vi "read data from lard.vi"() -> (0 "pos x":i16, 3 "distance":fxp<+/-,32,16>[](array[numeric]), 4 "pos y":i16, 6 "heading":i16)   [LabVIEW 2014]
uses:
  Robot Global Data.vi
panel:
  out "pos x 2":i16
  out "pos y 2":i16
  out "heading 2":sgl
  out "distance 2":fxp<+/-,32,16>[](array[numeric])
  in  "Boolean 2":bool
  in  "Boolean":bool
  out "Received Data":u8[](array[numeric])
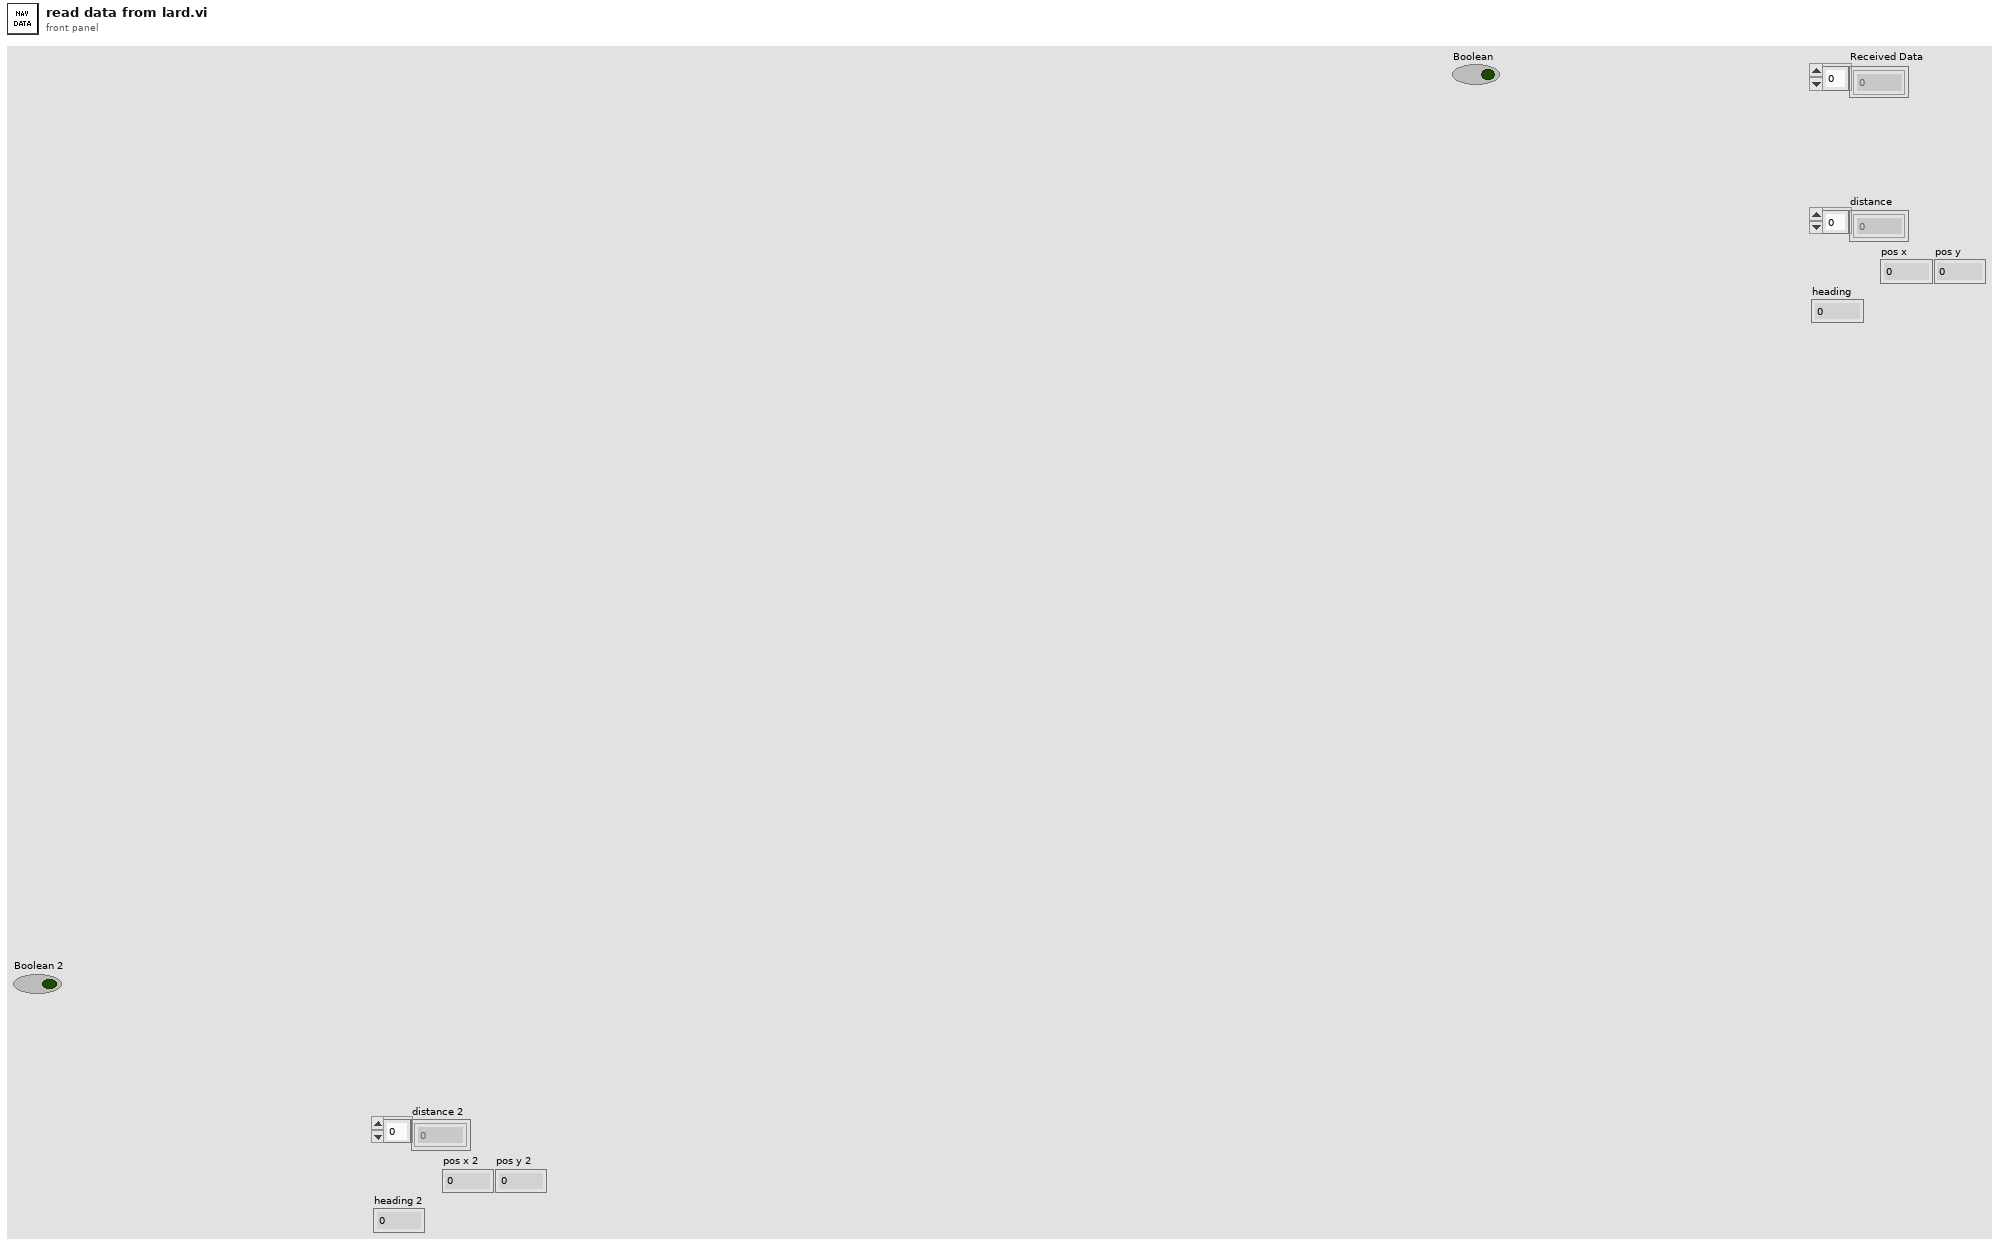
[diagram p1: front panel]
types:
  T1 = typedef "WPI_SerialPortRef.ctl" = cluster{"DevStatus":errorcluster, "Serial Port Name":refnum<visa-resource-name>}
  T2 = typedef "WPI_SPIDevRef.ctl" = cluster{"DevStatus":errorcluster, "Handle":i32, "Controller":T3, "SPI Bus":T4}
  T3 = typedef "FPGA_TypedefDigitalModule.ctl" = enum16{"Controller 1"}
  T4 = typedef "spi_bus.ctl" = enum16{"SPI On-Board, CS0", "SPI On-Board, CS1", "SPI On-Board, CS2", "SPI On-Board, CS3", "SPI MXP", "Invalid"}
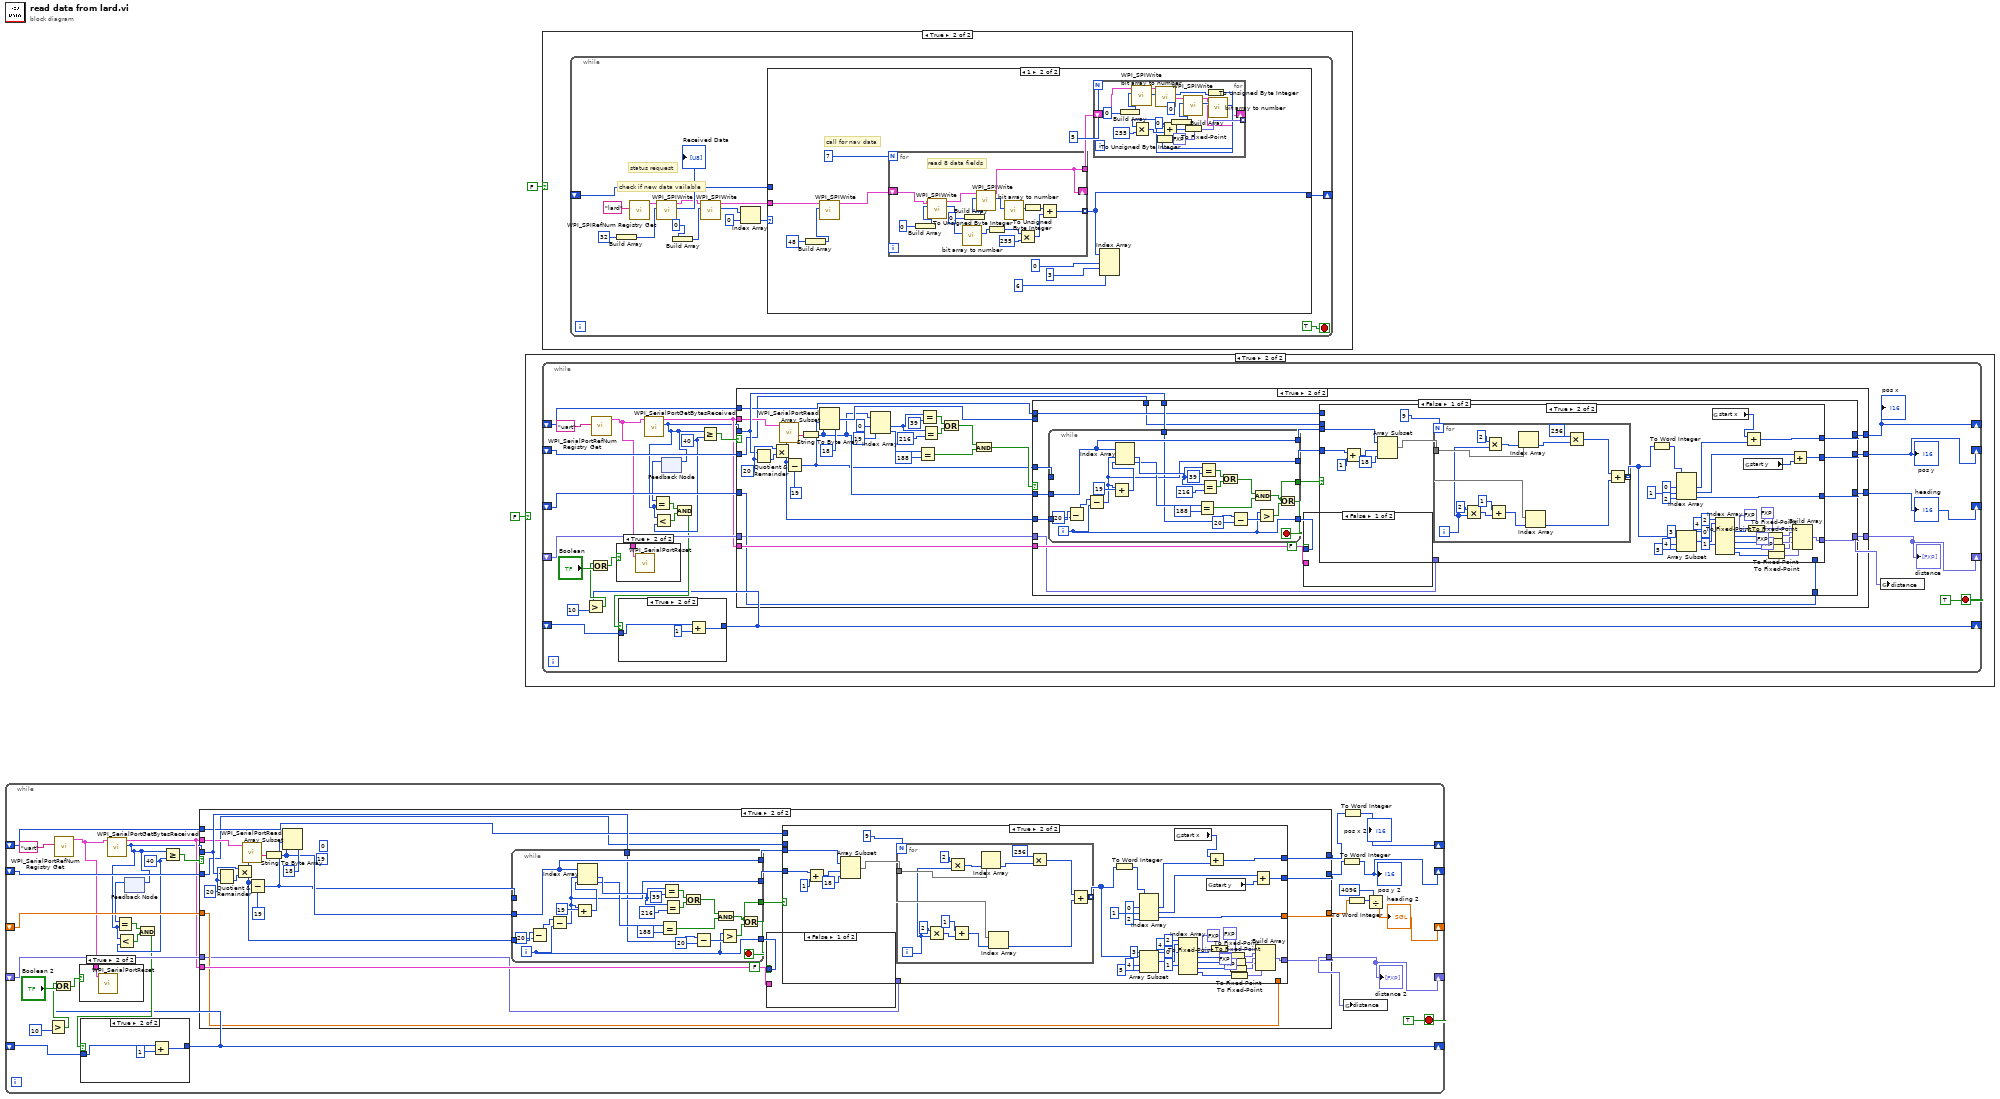
[diagram p0: block diagram]
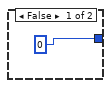
[diagram p2: hidden frame]
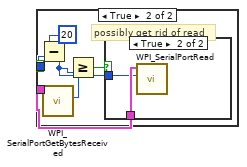
[diagram p6: hidden frame]
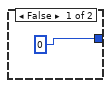
[diagram p9: hidden frame]
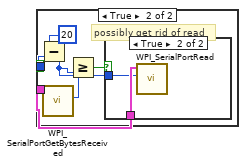
[diagram p13: hidden frame]
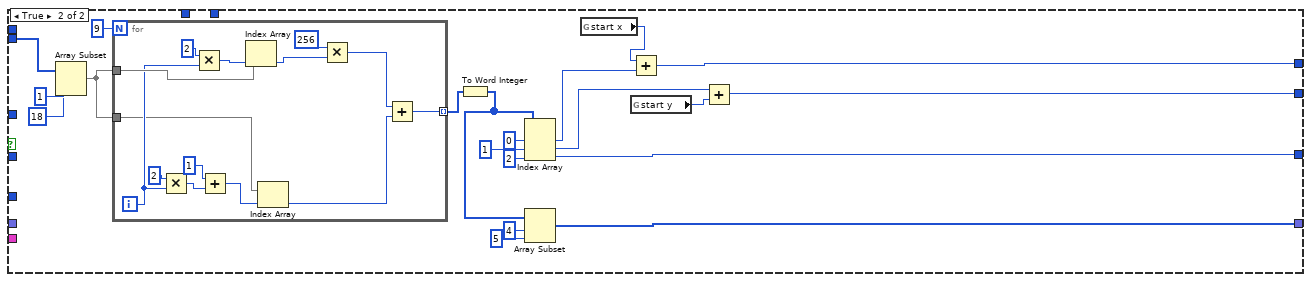
[diagram p15: hidden frame]
diagram:
  n1 = while {
    shift-right: [w9] -> _
    shift-left: _ -> [w29]
    shift-right: [w7] -> _
    shift-left: _ -> [w28]
    shift-right: [w3] -> _
    shift-left: _ -> [w27]
    shift-right: [w25] -> _
    shift-left: _ -> [w26]
    shift-right: [w11] -> _
    shift-left: _ -> [w14]
    stop <- TRUE stop-if-true
    w18 = u32 40 ("y")
    n2 = call <vilib>:"WPI_SerialPortRefNum Registry Get.vi"("refnum name"="uart") -> ("SerialPortRef"=w23:T1)  [unwired: 9 in, 1 out]
    n3 = call <vilib>:"WPI_SerialPortGetBytesReceived.vi"("SerialPortRef"=w23) -> ("Bytes at Port"=w19:u32, "SerialPortRef"=w24:T1)  [unwired: 8 in, 1 out]
    n4 = Less?(x=w19, y=w18) -> (x < y?=w16:bool)
    n5 = feedback-in #1(w19) -> ()
    n6 = feedback #1() -> (w20:u32)  [unwired: 1 in]
    n7 = Equal?(x=w20, y=w19) -> (x = y?=w17:bool)
    n8 = And(x=w17, y=w16) -> (x .and. y?=w15:bool)
    n9 = case shown="True" w15 {
      tunnel: [0 w34] -> w11
      tunnel: w14 -> [_ w36]
      frame False {
      }
      frame True {
        n10 = Add(x=w36, y=1) -> (x+y=w34:i32)
      }
    }
    n11 = Greater?(x=w11, y=10) -> (0:w12:bool)
    n12 = Or(x=w12, y="Boolean 2") -> (x .or. y?=w22:bool)
    n13 = case shown="True" w22 {
      tunnel: w23 -> [_ w37]
      frame False {
      }
      frame True {
        n14 = call <vilib>:"WPI_SerialPortReset.vi"("SerialPortRef"=w37) -> ()  [unwired: 9 in, 2 out]
      }
    }
    n15 = Greater Or Equal?(x=w19, y=w18) -> (x >= y?=w31:bool)
    n16 = case shown="True" w31 {
      tunnel: w24 -> [_ w51]
      tunnel: w19 -> [_ w52]
      tunnel: [w41 w62] -> w10
      tunnel: [w40 w61] -> w8
      tunnel: [w39 w60] -> w6
      tunnel: [w38 w59] -> w25
      tunnel: w29 -> [w41 w50]
      tunnel: w28 -> [w40 w49]
      tunnel: w27 -> [w39 w48]
      tunnel: w26 -> [w38 w47]
      tunnel: w24 -> [_ w55]
      frame False {
      }
      frame True {
        (unwired) 19 ("index")
        (unwired) 0 ("index")
        w58 = u32 20 ("y")
        n17 = Quotient & Remainder(x=w52, y=w58) -> (floor(x/y)=w57:u32)  [unwired: 1 out]
        n18 = Multiply(x=w58, y=w57) -> (x*y=w56:u32)
        n19 = call <vilib>:"WPI_SerialPortRead.vi"("Num Bytes to Read"=w56, "SerialPortRef"=w51) -> ("Buffer"=w65:string)  [unwired: 7 in, 2 out]
        n20 = Subtract(x=w56, y=u32 19) -> (x-y=w53:u32)
        n21 = String To Byte Array(string=w65) -> (unsigned byte array=w54:u8[])
        n22 = Array Subset(array=w54, index=w53, length=18) -> ()  [unwired: 1 out]
        n23 = while {
          tunnel: w54 -> [w146]
          tunnel: w56 -> [w138]
          tunnel: [w146] -> w46
          tunnel: [w139] -> w45
          tunnel: w53 -> [_]
          tunnel: [w143] -> w44
          tunnel: w52 -> [w142]
          tunnel: [w134] -> w42
          i -> [w139]
          stop <- w147 stop-if-true
          n24 = Subtract(x=w138, y=u32 20) -> (x-y=w136:u32)
          n25 = Subtract(x=w136, y=w139) -> (x-y=w143:u32)
          n26 = Add(x=w143, y=u32 19) -> (x+y=w144:u32)
          n27 = Index Array(array=w146, index #1=w143, index #2=w144) -> (element #1=w149:u8, element #2=w148:u8)
          n28 = Equal?(x=w148, y=u8 188) -> (x = y?=w150:bool)
          n29 = Equal?(x=w149, y=u8 39) -> (x = y?=w153:bool)
          n30 = Equal?(x=w149, y=u8 216) -> (x = y?=w152:bool)
          n31 = Or(x=w153, y=w152) -> (x .or. y?=w151:bool)
          n32 = Subtract(x=w142, y=u32 20) -> (x-y=w140:u32)
          n33 = And(x=w151, y=w150) -> (x .and. y?=w134:bool)
          n34 = Greater?(x=w139, y=w140) -> (0:w135:bool)
          n35 = Or(x=w134, y=w135) -> (x .or. y?=w147:bool)
        }
        n36 = case shown="False" FALSE {
          tunnel: w45 -> [_ w128]
          tunnel: w55 -> [_ w127]
          frame False {
          }
          frame True {
            # "possibly get rid of read"
            n37 = Subtract(x=20, y=w128) -> (x-y=w126:i32)
            n38 = call <vilib>:"WPI_SerialPortGetBytesReceived.vi"("SerialPortRef"=w127) -> ("Bytes at Port"=w130:u32)  [unwired: 8 in, 2 out]
            n39 = Greater Or Equal?(x=w130, y=w126) -> (x >= y?=w131:bool)
            n40 = case shown="True" w131 {
              tunnel: w127 -> [_ w133]
              tunnel: w126 -> [_ w132]
              frame False {
              }
              frame True {
                n41 = call <vilib>:"WPI_SerialPortRead.vi"("Num Bytes to Read"=w132, "SerialPortRef"=w133) -> ()  [unwired: 7 in, 3 out]
              }
            }
          }
        }
        n42 = case shown="True" w42 {
          tunnel: w46 -> [_ w103]
          tunnel: [w69 w98] -> w62
          tunnel: [w68 w97] -> w61
          tunnel: [w67 w96] -> w60
          tunnel: [w66 w70] -> w59
          tunnel: w44 -> [_ w93]
          tunnel: w50 -> [w69 _]
          tunnel: w49 -> [w68 _]
          tunnel: w48 -> [w67 _]
          tunnel: w47 -> [w66 _]
          frame False {
          }
          frame True {
            n43 = Add(x=w93, y=u32 1) -> (x+y=w102:u32)
            n44 = Array Subset(array=w103, index=w102, length=18) -> (w100:u8[])
            n45 = for {
              N: 9 -> [_]
              tunnel: w100 -> [w115]
              tunnel: [w113] -> w95 mode=indexing
              i -> [w114]
              n46 = Multiply(x=2, y=w114) -> (x*y=w122:i32)
              n47 = Multiply(x=2, y=w114) -> (x*y=w125:i32)
              n48 = Add(x=1, y=w122) -> (x+y=w120:i32)
              n49 = Index Array(array=w115, index=w125) -> (element=w118:u8)
              n50 = Index Array(array=w115, index=w120) -> (element=w116:u8)
              n51 = Multiply(x=i16 256, y=w118) -> (x*y=w117:i16)
              n52 = Add(x=w117, y=w116) -> (x+y=w113:i16)
            }
            n53 = To Word Integer(number=w95) -> (16bit integer=w94:i16[])
            n54 = Index Array(array=w94, index #1=0 ("index"), index #2=1 ("index"), index #3=2 ("index")) -> (element #1=w107:i16, element #2=w106:i16, element #3=w96:i16)
            n55 = Array Subset(array=w95, index=4, length=5) -> (w90:i16[])
            n56 = global read "Robot Global Data.vi" "start x"() -> (w109:u16)
            n57 = Index Array(array=w90, index #1=0 ("index"), index #2=1 ("index"), index #3=2 ("index"), index #4=3 ("index"), index #5=4 ("index")) -> (element #1=w88:i16, element #2=w85:i16, element #3=w84:i16, element #4=w81:i16, element #5=w80:i16)
            n58 = Add(x=w109, y=w107) -> (x+y=w98:u16)
            n59 = global read "Robot Global Data.vi" "start y"() -> (w108:u16)
            n60 = To Fixed-Point(fixed-point type=fxp<+/-,32,16> 8.0, number=w88) -> (fixed-point=w75:fxp<+/-,32,16>)
            n61 = To Fixed-Point(fixed-point type=fxp<+/-,32,16> 8.0, number=w85) -> (fixed-point=w74:fxp<+/-,32,16>)
            n62 = To Fixed-Point(fixed-point type=fxp<+/-,32,16> 8.0, number=w84) -> (fixed-point=w73:fxp<+/-,32,16>)
            n63 = To Fixed-Point(fixed-point type=fxp<+/-,32,16> 8.0, number=w81) -> (fixed-point=w72:fxp<+/-,32,16>)
            n64 = To Fixed-Point(fixed-point type=fxp<+/-,32,16> 8.0, number=w80) -> (fixed-point=w71:fxp<+/-,32,16>)
            n65 = Add(x=w106, y=w108) -> (x+y=w97:u16)
            n66 = Build Array(w75, w74, w73, w72, w71) -> (w70:fxp<+/-,32,16>[])
          }
        }
      }
    }
    "distance 2" <- w25
    n67 = To Word Integer(number=w8) -> (16bit integer=w7:i16)
    "pos y 2" <- w7
    n68 = To Word Integer(number=w10) -> (16bit integer=w9:i16)
    "pos x 2" <- w9
    n69 = global write "Robot Global Data.vi" "distance"(w25) -> ()
    n70 = To Word Integer(number=w6) -> (16bit integer=w5:i16)
    n71 = Divide(x=w5, y=i16 4096) -> (x/y=w3:dbl)
    "heading 2" <- w3
  }
  n72 = case shown="True" FALSE {
    frame False {
    }
    frame True {
      n73 = while {
        shift-right: [w178] -> _
        shift-left: _ -> [w175]
        shift-right: [w177] -> _
        shift-left: _ -> [w174]
        shift-right: [w176] -> _
        shift-left: _ -> [w173]
        shift-right: [w171] -> _
        shift-left: _ -> [w172]
        shift-right: [w157] -> _
        shift-left: _ -> [w160]
        stop <- TRUE stop-if-true
        w164 = u32 40 ("y")
        n74 = call <vilib>:"WPI_SerialPortRefNum Registry Get.vi"("refnum name"="uart") -> ("SerialPortRef"=w169:T1)  [unwired: 9 in, 1 out]
        n75 = call <vilib>:"WPI_SerialPortGetBytesReceived.vi"("SerialPortRef"=w169) -> ("Bytes at Port"=w165:u32, "SerialPortRef"=w170:T1)  [unwired: 8 in, 1 out]
        n76 = Less?(x=w165, y=w164) -> (x < y?=w162:bool)
        n77 = feedback-in #2(w165) -> ()
        n78 = feedback #2() -> (w166:u32)  [unwired: 1 in]
        n79 = Equal?(x=w166, y=w165) -> (x = y?=w163:bool)
        n80 = And(x=w163, y=w162) -> (x .and. y?=w161:bool)
        n81 = case shown="True" w161 {
          tunnel: [0 w183] -> w157
          tunnel: w160 -> [_ w185]
          frame False {
          }
          frame True {
            n82 = Add(x=w185, y=1) -> (x+y=w183:i32)
          }
        }
        n83 = Greater?(x=w157, y=10) -> (0:w158:bool)
        n84 = Or(x=w158, y="Boolean") -> (x .or. y?=w168:bool)
        n85 = case shown="True" w168 {
          tunnel: w169 -> [_ w186]
          frame False {
          }
          frame True {
            n86 = call <vilib>:"WPI_SerialPortReset.vi"("SerialPortRef"=w186) -> ()  [unwired: 9 in, 2 out]
          }
        }
        n87 = Greater Or Equal?(x=w165, y=w164) -> (x >= y?=w180:bool)
        n88 = case shown="True" w180 {
          tunnel: w170 -> [_ w195]
          tunnel: w165 -> [_ w196]
          tunnel: [w190 w219] -> w178
          tunnel: [w189 w218] -> w177
          tunnel: [w188 w217] -> w176
          tunnel: [w187 w216] -> w171
          tunnel: w175 -> [w190 w194]
          tunnel: w174 -> [w189 w193]
          tunnel: w173 -> [w188 w192]
          tunnel: w172 -> [w187 w191]
          tunnel: w170 -> [_ w199]
          frame False {
          }
          frame True {
            w215 = u32 20 ("y")
            n89 = Quotient & Remainder(x=w196, y=w215) -> (floor(x/y)=w214:u32)  [unwired: 1 out]
            n90 = Multiply(x=w215, y=w214) -> (x*y=w200:u32)
            n91 = call <vilib>:"WPI_SerialPortRead.vi"("Num Bytes to Read"=w200, "SerialPortRef"=w195) -> ("Buffer"=w222:string)  [unwired: 7 in, 2 out]
            n92 = Subtract(x=w200, y=u32 19) -> (x-y=w197:u32)
            n93 = String To Byte Array(string=w222) -> (unsigned byte array=w198:u8[])
            n94 = Array Subset(array=w198, index=w197, length=18) -> (w201:u8[])
            n95 = Index Array(array=w198, index #1=0 ("index"), index #2=19 ("index")) -> (element #1=w210:u8, element #2=w208:u8)
            n96 = Equal?(x=w208, y=u8 188) -> (x = y?=w203:bool)
            n97 = Equal?(x=w210, y=u8 39) -> (x = y?=w206:bool)
            n98 = Equal?(x=w210, y=u8 216) -> (x = y?=w205:bool)
            n99 = Or(x=w206, y=w205) -> (x .or. y?=w204:bool)
            n100 = And(x=w204, y=w203) -> (x .and. y?=w202:bool)
            n101 = case shown="False" w202 {
              tunnel: [w237 w341] -> w219
              tunnel: [w236 w340] -> w218
              tunnel: [w235 w339] -> w217
              tunnel: [w234 w338] -> w216
              tunnel: w201 -> [_ w337]
              tunnel: w198 -> [w240 _]
              tunnel: w200 -> [w239 _]
              tunnel: w199 -> [w232 _]
              tunnel: w197 -> [w231 _]
              tunnel: w196 -> [w229 _]
              tunnel: w194 -> [w227 _]
              tunnel: w193 -> [w226 _]
              tunnel: w192 -> [w225 _]
              tunnel: w191 -> [w224 _]
              frame False {
                n102 = while {
                  tunnel: w240 -> [w321]
                  tunnel: w239 -> [w313]
                  tunnel: [w321] -> w238
                  tunnel: [w314] -> w233
                  tunnel: w231 -> [_]
                  tunnel: [w318] -> w230
                  tunnel: w229 -> [w317]
                  tunnel: [w309] -> w223
                  i -> [w314]
                  stop <- w322 stop-if-true
                  n103 = Subtract(x=w313, y=u32 20) -> (x-y=w311:u32)
                  n104 = Subtract(x=w311, y=w314) -> (x-y=w318:u32)
                  n105 = Add(x=w318, y=u32 19) -> (x+y=w319:u32)
                  n106 = Index Array(array=w321, index #1=w318, index #2=w319) -> (element #1=w324:u8, element #2=w323:u8)
                  n107 = Equal?(x=w323, y=u8 188) -> (x = y?=w325:bool)
                  n108 = Equal?(x=w324, y=u8 39) -> (x = y?=w328:bool)
                  n109 = Equal?(x=w324, y=u8 216) -> (x = y?=w327:bool)
                  n110 = Or(x=w328, y=w327) -> (x .or. y?=w326:bool)
                  n111 = Subtract(x=w317, y=u32 20) -> (x-y=w315:u32)
                  n112 = And(x=w326, y=w325) -> (x .and. y?=w309:bool)
                  n113 = Greater?(x=w314, y=w315) -> (0:w310:bool)
                  n114 = Or(x=w309, y=w310) -> (x .or. y?=w322:bool)
                }
                n115 = case shown="False" FALSE {
                  tunnel: w233 -> [_ w303]
                  tunnel: w232 -> [_ w302]
                  frame False {
                  }
                  frame True {
                    # "possibly get rid of read"
                    n116 = Subtract(x=20, y=w303) -> (x-y=w301:i32)
                    n117 = call <vilib>:"WPI_SerialPortGetBytesReceived.vi"("SerialPortRef"=w302) -> ("Bytes at Port"=w305:u32)  [unwired: 8 in, 2 out]
                    n118 = Greater Or Equal?(x=w305, y=w301) -> (x >= y?=w306:bool)
                    n119 = case shown="True" w306 {
                      tunnel: w302 -> [_ w308]
                      tunnel: w301 -> [_ w307]
                      frame False {
                      }
                      frame True {
                        n120 = call <vilib>:"WPI_SerialPortRead.vi"("Num Bytes to Read"=w307, "SerialPortRef"=w308) -> ()  [unwired: 7 in, 3 out]
                      }
                    }
                  }
                }
                n121 = case shown="True" w223 {
                  tunnel: w238 -> [_ w278]
                  tunnel: [w244 w273] -> w237
                  tunnel: [w243 w272] -> w236
                  tunnel: [w242 w271] -> w235
                  tunnel: [w241 w245] -> w234
                  tunnel: w230 -> [_ w268]
                  tunnel: w227 -> [w244 _]
                  tunnel: w226 -> [w243 _]
                  tunnel: w225 -> [w242 _]
                  tunnel: w224 -> [w241 _]
                  frame False {
                  }
                  frame True {
                    n122 = Add(x=w268, y=u32 1) -> (x+y=w277:u32)
                    n123 = Array Subset(array=w278, index=w277, length=18) -> (w275:u8[])
                    n124 = for {
                      N: 9 -> [_]
                      tunnel: w275 -> [w290]
                      tunnel: [w288] -> w270 mode=indexing
                      i -> [w289]
                      n125 = Multiply(x=2, y=w289) -> (x*y=w297:i32)
                      n126 = Multiply(x=2, y=w289) -> (x*y=w300:i32)
                      n127 = Add(x=1, y=w297) -> (x+y=w295:i32)
                      n128 = Index Array(array=w290, index=w300) -> (element=w293:u8)
                      n129 = Index Array(array=w290, index=w295) -> (element=w291:u8)
                      n130 = Multiply(x=i16 256, y=w293) -> (x*y=w292:i16)
                      n131 = Add(x=w292, y=w291) -> (x+y=w288:i16)
                    }
                    n132 = To Word Integer(number=w270) -> (16bit integer=w269:i16[])
                    n133 = Index Array(array=w269, index #1=0 ("index"), index #2=1 ("index"), index #3=2 ("index")) -> (element #1=w282:i16, element #2=w281:i16, element #3=w271:i16)
                    n134 = Array Subset(array=w270, index=4, length=5) -> (w265:i16[])
                    n135 = global read "Robot Global Data.vi" "start x"() -> (w284:u16)
                    n136 = Index Array(array=w265, index #1=0 ("index"), index #2=1 ("index"), index #3=2 ("index"), index #4=3 ("index"), index #5=4 ("index")) -> (element #1=w263:i16, element #2=w260:i16, element #3=w259:i16, element #4=w256:i16, element #5=w255:i16)
                    n137 = Add(x=w284, y=w282) -> (x+y=w273:u16)
                    n138 = global read "Robot Global Data.vi" "start y"() -> (w283:u16)
                    n139 = To Fixed-Point(fixed-point type=fxp<+/-,32,16> 8.0, number=w263) -> (fixed-point=w250:fxp<+/-,32,16>)
                    n140 = To Fixed-Point(fixed-point type=fxp<+/-,32,16> 8.0, number=w260) -> (fixed-point=w249:fxp<+/-,32,16>)
                    n141 = To Fixed-Point(fixed-point type=fxp<+/-,32,16> 8.0, number=w259) -> (fixed-point=w248:fxp<+/-,32,16>)
                    n142 = To Fixed-Point(fixed-point type=fxp<+/-,32,16> 8.0, number=w256) -> (fixed-point=w247:fxp<+/-,32,16>)
                    n143 = To Fixed-Point(fixed-point type=fxp<+/-,32,16> 8.0, number=w255) -> (fixed-point=w246:fxp<+/-,32,16>)
                    n144 = Add(x=w281, y=w283) -> (x+y=w272:u16)
                    n145 = Build Array(w250, w249, w248, w247, w246) -> (w245:fxp<+/-,32,16>[])
                  }
                }
              }
              frame True {
                n146 = Array Subset(array=w337, index=1, length=18) -> (w334:u8[])
                n147 = for {
                  N: 9 -> [_]
                  tunnel: w334 -> [w363]
                  tunnel: w334 -> [w357]
                  tunnel: [w352] -> w333 mode=indexing
                  i -> [w362]
                  n148 = Multiply(x=2, y=w362) -> (x*y=w360:i32)
                  n149 = Multiply(x=2, y=w362) -> (x*y=w365:i32)
                  n150 = Add(x=1, y=w360) -> (x+y=w358:i32)
                  n151 = Index Array(array=w363, index=w365) -> (element=w355:u8)
                  n152 = Index Array(array=w357, index=w358) -> (element=w353:u8)
                  n153 = Multiply(x=i16 256, y=w355) -> (x*y=w354:i16)
                  n154 = Add(x=w354, y=w353) -> (x+y=w352:i16)
                }
                n155 = To Word Integer(number=w333) -> (16bit integer=w332:i16[])
                n156 = Index Array(array=w332, index #1=0 ("index"), index #2=1 ("index"), index #3=2 ("index")) -> (element #1=w345:i16, element #2=w344:i16, element #3=w339:i16)
                n157 = Array Subset(array=w332, index=4, length=5) -> (w338:i16[])
                n158 = global read "Robot Global Data.vi" "start x"() -> (w347:u16)
                n159 = Add(x=w347, y=w345) -> (x+y=w341:u16)
                n160 = global read "Robot Global Data.vi" "start y"() -> (w346:u16)
                n161 = Add(x=w344, y=w346) -> (x+y=w340:u16)
              }
            }
          }
        }
        "pos x" <- w178
        "pos y" <- w177
        "heading" <- w176
        "distance" <- w171
        n162 = global write "Robot Global Data.vi" "distance"(w171) -> ()
      }
    }
  }
  n163 = case shown="True" FALSE {
    frame False {
    }
    frame True {
      n164 = while {
        shift-right: [w377] -> _
        shift-left: _ -> [w376]
        stop <- TRUE stop-if-true
        # "status request"
        # "check if new data vailable"
        n165 = Build Array(32) -> (w373:i32[])
        n166 = call <vilib>:"WPI_SPIRefNum Registry Get.vi"("refnum name"="lard") -> ("SPIDevRef"=w380:T2)  [unwired: 9 in, 1 out]
        n167 = call <vilib>:"WPI_SPIWrite.vi"("Data To Send"=w373, "SPIDevRef"=w380) -> ("Received Data"=→"Received Data":u8[], "SPIDevRef"=w369:T2)  [unwired: 7 in, 1 out]
        n168 = Build Array(0 ("Num to Read")) -> (w366:i32[])
        n169 = call <vilib>:"WPI_SPIWrite.vi"("Data To Send"=w366, "SPIDevRef"=w369) -> ("Received Data"=w367:u8[], "SPIDevRef"=w368:T2)  [unwired: 7 in, 1 out]
        n170 = Index Array(array=w367, index=0) -> (element=w371:u8)
        n171 = case shown="1" w371 {
          tunnel: w368 -> [_ w391]
          tunnel: [w381 w389] -> w377
          tunnel: w376 -> [w381 _]
          frame 0, Default {
          }
          frame 1 {
            # "call for nav data"
            n172 = Build Array(48) -> (w384:i32[])
            n173 = call <vilib>:"WPI_SPIWrite.vi"("Data To Send"=w384, "SPIDevRef"=w391) -> ("SPIDevRef"=w383:T2)  [unwired: 7 in, 2 out]
            n174 = for {
              N: 7 -> [_]
              tunnel: [w424] -> w389 mode=indexing
              tunnel: [w411] -> w382
              shift-right: [w411] -> _
              shift-left: w383 -> [w418]
              # "read 8 data fields"
              n175 = Build Array(0 ("Num to Read")) -> (w416:i32[])
              n176 = call <vilib>:"WPI_SPIWrite.vi"("Data To Send"=w416, "SPIDevRef"=w418) -> ("Received Data"=w419:u8[], "SPIDevRef"=w413:T2)  [unwired: 7 in, 1 out]
              n177 = call "bit array to number.vi"("bit array"=w419) -> ("Numeric"=w423:i32)  [unwired: 10 in]
              n178 = Build Array(0 ("Num to Read")) -> (w414:i32[])
              n179 = call <vilib>:"WPI_SPIWrite.vi"("Data To Send"=w414, "SPIDevRef"=w413) -> ("Received Data"=w412:u8[], "SPIDevRef"=w411:T2)  [unwired: 7 in, 1 out]
              n180 = To Unsigned Byte Integer(number=w423) -> (unsigned 8bit integer=w422:u8)
              n181 = call "bit array to number.vi"("bit array"=w412) -> ("Numeric"=w421:i32)  [unwired: 10 in]
              n182 = Multiply(x=w422, y=u16 255) -> (x*y=w425:u16)
              n183 = To Unsigned Byte Integer(number=w421) -> (unsigned 8bit integer=w420:u8)
              n184 = Add(x=w420, y=w425) -> (x+y=w424:u16)
            }
            n185 = for {
              N: 5 -> [_]
              tunnel: [w410] -> _ mode=indexing
              shift-right: [w393] -> _
              shift-left: w382 -> [w399]
              (unwired) 0 ("Num to Read")
              n186 = Build Array(0 ("Num to Read")) -> (w401:i32[])
              n187 = call <vilib>:"WPI_SPIWrite.vi"("Data To Send"=w401, "SPIDevRef"=w399) -> ("Received Data"=w398:u8[], "SPIDevRef"=w395:T2)  [unwired: 7 in, 1 out]
              n188 = call "bit array to number.vi"("bit array"=w398) -> ("Numeric"=w405:i32)  [unwired: 10 in]
              n189 = Build Array(0 ("Num to Read")) -> (w396:i32[])
              n190 = call <vilib>:"WPI_SPIWrite.vi"("Data To Send"=w396, "SPIDevRef"=w395) -> ("Received Data"=w394:u8[], "SPIDevRef"=w393:T2)  [unwired: 7 in, 1 out]
              n191 = To Unsigned Byte Integer(number=w405) -> (unsigned 8bit integer=w404:u8)
              n192 = Multiply(x=w404, y=255) -> (x*y=w408:i32)
              n193 = call "bit array to number.vi"("bit array"=w394) -> ("Numeric"=w402:i32)  [unwired: 10 in]
              n194 = To Unsigned Byte Integer(number=w402) -> (unsigned 8bit integer=w403:u8)
              n195 = Add(x=w403, y=w408) -> (x+y=w407:i32)
              n196 = To Fixed-Point(fixed-point type=fxp<+/-,32,16> 8.0, number=w407) -> (fixed-point=w410:fxp<+/-,32,16>)
            }
            n197 = Index Array(array=w389, index #1=0 ("index"), index #2=3 ("index"), index #3=6 ("index")) -> ()  [unwired: 3 out]
          }
        }
      }
    }
  }
